vi "PDC_GetResolution.vi"(8 "error in (no error)":errorcluster, 10 "ChildNo":u32, 11 "DeviceNo":u32) -> (0 "error out":errorcluster, 1 "Height":u32, 2 "Width":u32, 3 "ReturnValue":u32, 4 "ErrorCode":u32)   [LabVIEW 2015]
doc: "This VI retrieves the resolution of the specified child device."
uses:
  PDCLIB.dll
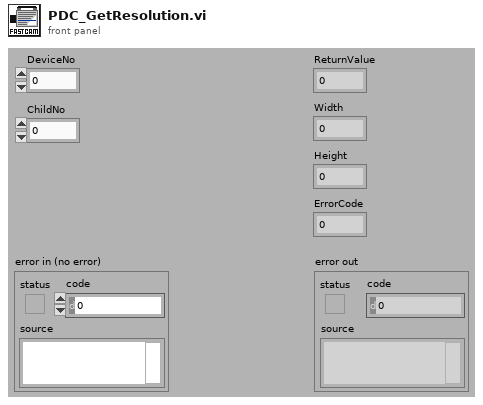
[diagram p1: front panel]
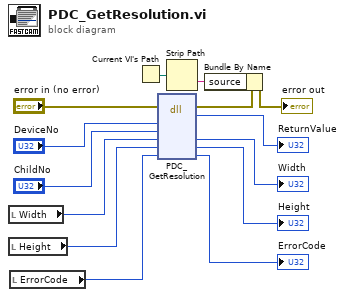
[diagram p0: block diagram]
diagram:
  n1 = local read "Width"() -> (w7:u32)
  n2 = local read "Height"() -> (w6:u32)
  n3 = local read "ErrorCode"() -> (w11:u32)
  n4 = Current VI's Path() -> (path=w3:path)
  n5 = dll-call lib="PDCLIB.dll" fn="PDC_GetResolution"(error in="error in (no error)", "nDeviceNo"="DeviceNo", "nChildNo"="ChildNo", "pWidth"=w7, "pHeight"=w6, "pErrorCode"=w11) -> (error out=w2:errorcluster, "return type"=→"ReturnValue":u32, "pWidth"=→"Width":u32, "pHeight"=→"Height":u32, "pErrorCode"=→"ErrorCode":u32)  [unwired: 4 in, 1 out]
  n6 = Strip Path(path=w3) -> (name=w4:string)  [unwired: 1 out]
  n7 = Bundle By Name(cluster=w2, "source"=w4) -> (→"error out":errorcluster)
